vi "GetNumCamFramesv2.vi"(9 "Digital Waveform Graph":digitalwaveform[](array[waveform])) -> (3 "Numeric":i32)   [LabVIEW 2015]
uses:
  <vilib>/Waveform/DWDTOps.llb/DWDT Digital to Boolean Array.vi
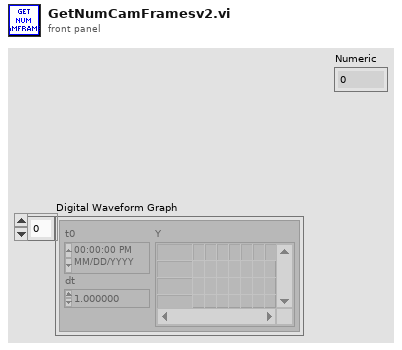
[diagram p1: front panel]
types:
  T1 = typedef "LVRectTypeDef.ctl" = cluster{"Left":i16, "Top":i16, "Right":i16, "Bottom":i16}
  T2 = cluster{"Xpixels":i32, "Vxminref":dbl, "Vxmaxref":dbl, "P":dbl, "Ypixels":i32, "Vyminref":dbl, "Vymaxref":dbl, "srate":sgl, "sAOxy":i32, "timeout":dbl, "type":string, "date":string, "time":string, "Colormap":u16, "Drawing Mode":u16, "Scanning Mode":u16, "square pixels":bool, "square matrix":bool, "Xpixels Img":i32, "Vx-min Img":dbl, "VX-max Img":dbl, "Ypixels Img":i32, "Vy-min Img":dbl, "Vy-max Img ":dbl, "Angle Img":dbl, "autoshutter":bool, "finite":bool, "cont":bool, "wavdet":bool, "measpoints":i32, "avpp":i32, "bufferAO":i32, "bufferAI":i32, "starttick":u32, "waveform":path, "Vx-ref":dbl, "Vy-ref":dbl, "refreshrate":dbl, "refreshbuffer":i32, "tt_cycles":i32, "motorref":refnum<k7>, "mirrorswitch":refnum<k7>, "sample mode":i32, "maxbufferAI":i32, "srateAODO":sgl, "bin":sgl, "Pel":sgl, "Angle draw":dbl, "srate Img":sgl, "ROIimg_plotbounds":T1, "auto OD":bool, "ODfilt":u16, "aAI":i32[], "aCI":i32[], "aAO":u32[], "aDO":u32[], "refwfsize":dbl, "Lifetime":bool, "Vz-Img":dbl, "Vz-ref":dbl, "Vz-reset":dbl, "AIoverride":bool, "aAS":u32[], "XYZstart":dbl[], "External 100KHz Clock?":bool}
  T3 = typedef "XYZStage.lvlib/XYZStage Configuration.ctl" = cluster{"VISA resource name":refnum<visa-resource-name>, "Timeout (3sec)":u32}
  T4 = cluster{"StageS":i32, "StageL":i32, "currmeas data dir":path, "image OD":u16, "contour OD":u16, "point OD":u16, "AOlines":tag[], "AIlines":tag[], "CI lines":tag[], "DO lines":tag[], "AO names":string[], "CI names":string[], "AI names":string[], "DO names":string[], "CIextensions":string[], "AIextensions":string[], "Voltage to Ygalvo":i32, "Voltage to Xgalvo":i32, "Voltage to patch":i32, "640 shutter":i32, "2P shutter":i32, "LT timestamp":u32, "Vp":i32, "Ip":i32, "camera trigger":i32, "master data dir":path, "voltage to Zpos":i32, "Vto2P":i32, "640 AO":i32, "488 AO":i32, "532 AO":i32, "640TTL":u32, "488TTL":u32, "532TTL":u32, "Device 1 sampleclock out":tag, "Device 1 Starttrigger out":tag, "Device 2 sampleclock in":tag, "Device 2 StartTrigger in ":tag, "2PODTTL":u32, "488 shutter":u32, "LCVR red":u32, "LCVR blue":u32, "Sutter Stage Config":T3, "Device 1 ext sampleclock in (100Khz)":tag}
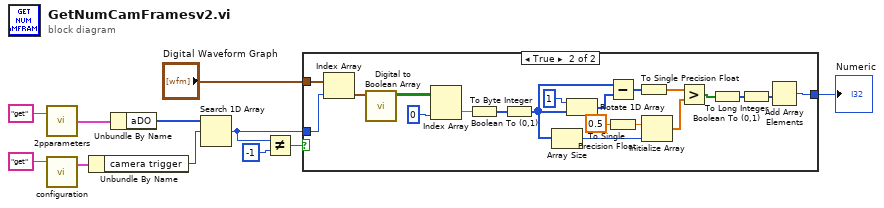
[diagram p0: block diagram]
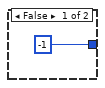
[diagram p2: hidden frame]
diagram:
  n1 = call "2pparameters.vi"("command"="get") -> ("params out"=w7:T2)  [unwired: 1 in]
  n2 = call "configuration.vi"("command"="get") -> ("config out"=w9:T4)  [unwired: 2 in, 1 out]
  n3 = Unbundle By Name(w9) -> ("camera trigger"=w5:i32)
  n4 = Unbundle By Name(w7) -> ("aDO"=w6:u32[])
  n5 = Search 1D Array(1D array=w6, element=w5) -> (index of element=w2:i32)  [unwired: 1 in]
  n6 = Not Equal?(x=w2, y=-1) -> (x != y?=w3:bool)
  n7 = case shown="True" w3 {
    tunnel: "Digital Waveform Graph" -> [_ w31]
    tunnel: w2 -> [_ w32]
    tunnel: [-1 w13] -> w1
    frame False {
    }
    frame True {
      n8 = Index Array(array=w31, index=w32) -> (element=w30:digitalwaveform)
      n9 = call-poly <vilib>:"Digital to Boolean Array.vi"("digital waveform"=w30) -> ("boolean array"=w29:bool[][])  [unwired: 9 in, 1 out]
      n10 = Index Array(array=w29, index (col)=0) -> (element=w26:bool[])  [unwired: 1 in]
      n11 = Boolean To (0,1)(Boolean=w26) -> (0, 1=w25:i16[])
      n12 = To Byte Integer(number=w25) -> (8bit integer=w22:i8[])
      n13 = Array Size(array=w22) -> (size(s)=w21:i32)
      n14 = Rotate 1D Array(1:w22, 2:1 ("n")) -> (0:w24:i8[])
      n15 = Subtract(x=w22, y=w24) -> (x-y=w23:i8[])
      n16 = To Single Precision Float(number=0.5 ("element")) -> (single precision float=w15:sgl)
      n17 = To Single Precision Float(number=w23) -> (single precision float=w16:sgl[])
      n18 = Initialize Array(w15, w21) -> (w19:sgl[])
      n19 = Greater?(x=w16, y=w19) -> (0:w18:bool[])
      n20 = Boolean To (0,1)(Boolean=w18) -> (0, 1=w17:i16[])
      n21 = To Long Integer(number=w17) -> (32bit integer=w14:i32[])
      n22 = Add Array Elements(numeric array=w14) -> (sum=w13:i32)
    }
  }
  "Numeric" <- w1
